vi "test_launchBrokenTaskShouldReturnError1003.vi"(11 "Test Case In":refnum<class "TaskControllerTests.lvclass">) -> (0 "error out":errorcluster, 3 "Test Case Out":refnum<class "TaskControllerTests.lvclass">)   [LabVIEW 2023, in "TaskControllerTests.lvclass"]
uses:
  TaskControllerTests.lvclass
  <vilib>/Astemes/LUnit/Test Case.lvclass/Test Case.ctl
  <vilib>/Astemes/LUnit/Palette/Pass If Error.vi
  <vilib>/Astemes/LUnit/Palette/Advanced Assertions/Pass If Specific Error.vi/d0e67a5c-31db-4060-a993-98defbf94426.vi
  <vilib>/Astemes/LUnit/Palette/Fail.vi
  <vilib>/Astemes/LUnit/Core/LUnit Test Case/Private/Append Fail Result.vi
  <vilib>/Astemes/LUnit/Core/LUnit Test Case/Private/Append Pass Result.vi
  <vilib>/Astemes/LUnit/Core/LUnit Test Case/Private/Run In UI.vi
  <vilib>/Utility/error.llb/Clear Errors.vi
  TaskMock/TaskMock.lvclass
  <vilib>/Comparison/Equal/Equal Functor/Equal Functor.lvclass
  TaskControllerTests.lvclass/TaskControllerTests.ctl
  source/TaskController/TaskController.lvclass
  <vilib>/Astemes/LUnit/Palette/Advanced Assertions/LUnit Advanced Assertions.lvlib
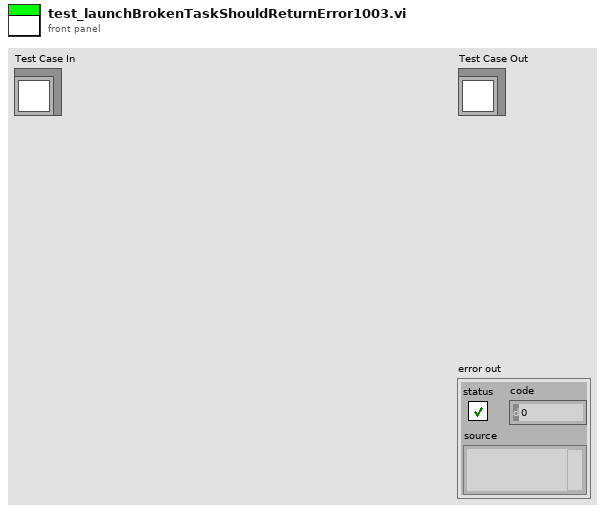
[diagram p1: front panel]
types:
  T1 = enum16{"ValidTask", "BrokenTask", "InvalidConnectorPaneTask"}
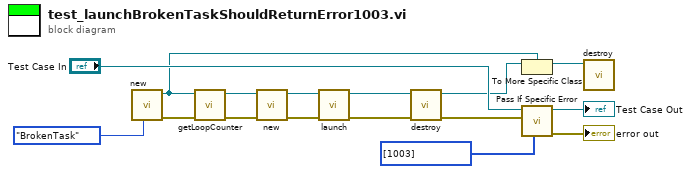
[diagram p0: block diagram]
diagram:
  n1 = call "new.vi"("taskType"=T1."BrokenTask") -> ("error out"=w6:errorcluster, "TaskMock out"=w9:refnum<class "TaskMock.lvclass">)  [unwired: 9 in]
  n2 = call "getLoopCounter.vi"("error in (no error)"=w6, "TaskMock in"=w9) -> ("error out"=w5:errorcluster, "TaskMock out"=w11:refnum<class "TaskMock.lvclass">)  [unwired: 7 in, 1 out]
  n3 = call "new.vi"("error in (no error)"=w5, "task"=w11) -> ("error out"=w12:errorcluster, "TaskController out"=w13:refnum<class "TaskController.lvclass">)  [unwired: 8 in]
  n4 = call "launch.vi"("error in (no error)"=w12, "TaskController in"=w13) -> ("error out"=w3:errorcluster, "TaskController out"=w10:refnum<class "TaskController.lvclass">)  [unwired: 8 in]
  n5 = call "destroy.vi"("error in (no error)"=w3, "TaskController in"=w10) -> ("error out"=w1:errorcluster, "taskResult"=w8:refnum<class "ITask.lvclass">)  [unwired: 8 in]
  n6 = To More Specific Class(target class=w9, reference=w8) -> (specific class reference=w7:refnum<class "TaskMock.lvclass">)  [unwired: 1 in, 1 out]
  n7 = call <vilib>:"Pass If Specific Error.vi"("Error Codes"=i32[] [1003], "Assert error"=w1, "LUnit Test Case In"="Test Case In") -> ("error out"=→"error out":errorcluster, "LUnit Test Case Out"=→"Test Case Out":refnum<class "TaskControllerTests.lvclass">)  [unwired: 7 in]
  n8 = call "destroy.vi"("TaskMock in"=w7) -> ()  [unwired: 10 in, 1 out]
